vi "Dresden New Recipe.vi"() -> ()   [LabVIEW 2009]
panel:
  in  "New_recipe":bool
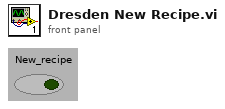
[diagram p1: front panel]
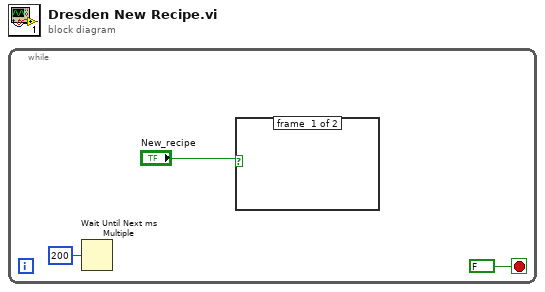
[diagram p0: block diagram]
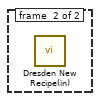
[diagram p2: hidden frame]
diagram:
  n1 = while {
    stop <- FALSE stop-if-true
    n2 = Wait Until Next ms Multiple(millisecond multiple=u32 200) -> ()  [unwired: 1 out]
    n3 = case shown="True" "New_recipe" {
      frame #0 {
      }
      frame #1 {
        n4 = call "Dresden New Recipe(in).vi"() -> ()  [unwired: 2 out]
      }
    }
  }
